vi "Post action.vi"(6 "Index":i32=41, 8 "error in (no error)":errorcluster, 9 "PostAction":T1, 11 "SweepControl":refnum<class "SMO.SweepControl.lvclass">) -> (0 "error out":errorcluster, 3 "SweepControl":refnum<class "SMO.SweepControl.lvclass">)   [LabVIEW 2019, in "SMO.SweepControl.lvclass"]
uses:
  SMO.SweepControl.lvclass
  <userlib>/LevyLab/Instrument Framework/Instrument Types/Cryostat/Instrument.Cryostat.lvclass
  SMO.Control Experiment/SMO.Control Experiment.lvclass
  Control Experiment SM/Control Experiment SM.lvclass
  C:/Program Files (x86)/National Instruments/LabVIEW 2019/user.lib/LevyLab/Instrument Framework/SMOs/Instrument/Instrument.lvclass
  C:/Program Files (x86)/National Instruments/LabVIEW 2019/vi.lib/JKI/JKI SMO/SMO/SMO.lvclass
  Typedefs/Enum - PostAction.ctl
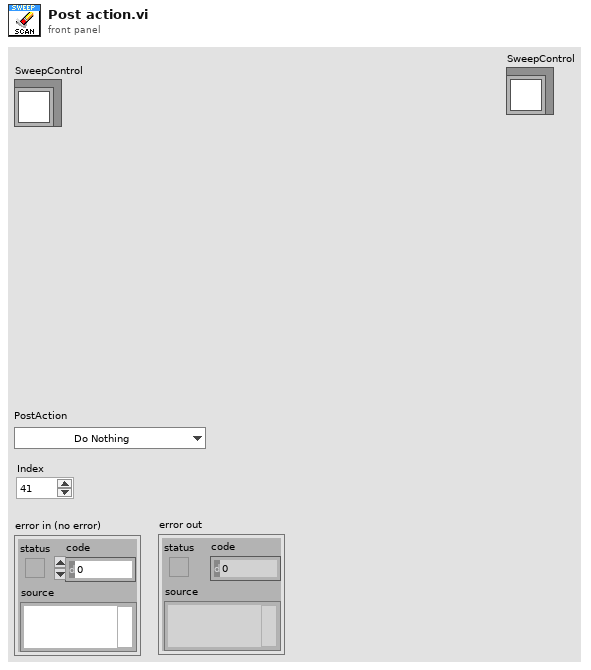
[diagram p1: front panel]
types:
  T1 = typedef "SMO.SweepControl.lvclass/Enum - PostAction.ctl" = enum16{"Do Nothing", "Wait (time)", "Wait (Temperature)", "Wait (<T ; B sweep)", "Wait (Magnet)"}
  T2 = typedef "SMO.SweepControl.lvclass/Cluster - ScanParamters.ctl" = cluster{"Start":dbl, "End":dbl, "Step":dbl, "Rate":dbl, "Waveform type":enum16{"linear", "triangle", "power"}, "wait (ms or K)":dbl, "Address":string, "channel":i32}
  T3 = typedef "SMO.Control Experiment.lvclass/Instruments--cluster.ctl" = cluster{"Lockin":refnum<class "Instrument.Lockin.lvclass">, "Temperature":refnum<class "Instrument.Cryostat.lvclass">, "Magnet":refnum<class "Instrument.Cryostat.lvclass">, "Rotator":refnum<class "Instrument.Cryostat.lvclass">, "Level":refnum<class "Instrument.Cryostat.lvclass">, "C Bridge":refnum<class "Instrument.CBridge.lvclass">, "Optical Delay Line":refnum<class "Instrument.DelayLine.lvclass">, "Strain Cell":refnum<class "Instrument.Strain.lvclass">, "VNA":refnum<class "Instrument.VNA.lvclass">, "Voltage Source":refnum<class "Instrument.VSource.lvclass">, "KH7008":refnum<class "Instrument.KH7008.lvclass">[]}
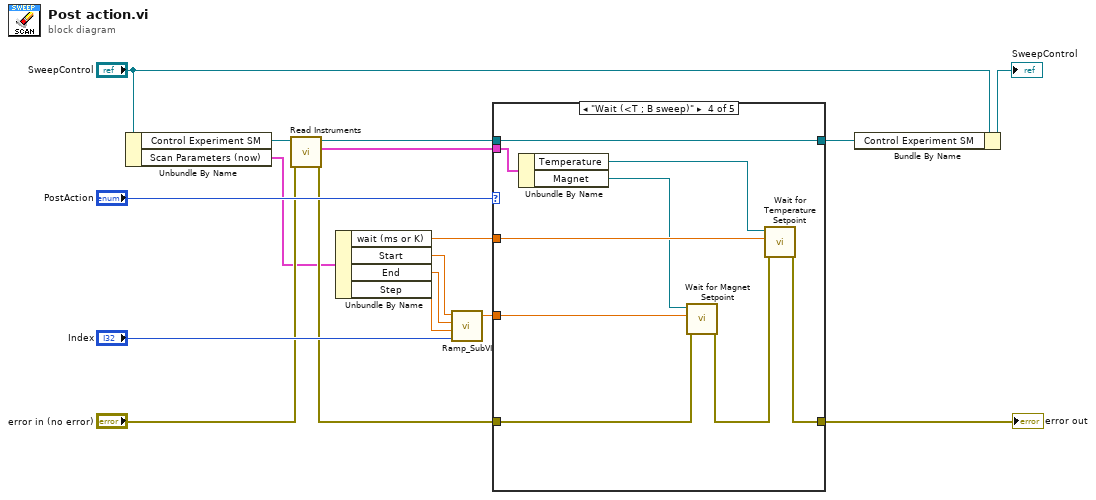
[diagram p0: block diagram]
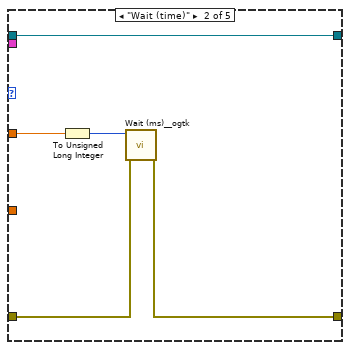
[diagram p3: hidden frame]
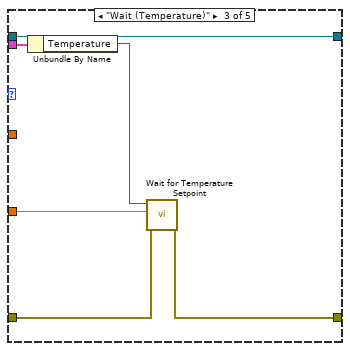
[diagram p4: hidden frame]
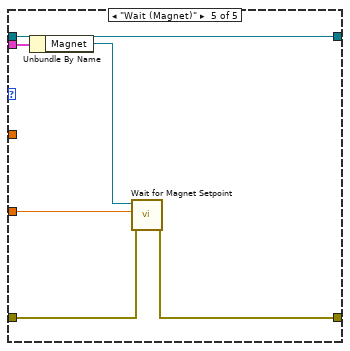
[diagram p5: hidden frame]
diagram:
  n1 = Unbundle By Name("SweepControl") -> ("Control Experiment SM"=w9:refnum<class "Control Experiment SM.lvclass">, "Scan Parameters (now)"=w1:T2)
  n2 = call "Read Instruments.vi"("error in (no error)"="error in (no error)", "Control Experiment"=w9) -> ("error out"=w6:errorcluster, "Instruments"=w8:T3, "Control Experiment out"=w2:refnum<class "SMO.Control Experiment.lvclass">)  [unwired: 7 in]
  n3 = Unbundle By Name(w1) -> ("wait (ms or K)"=w11:dbl, "Start"=w14:dbl, "End"=w13:dbl, "Step"=w12:dbl)
  n4 = call <userlib>:"Ramp_SubVI.vi"("index"="Index", "step"=w12, "end"=w13, "start"=w14) -> ("Numeric"=w16:dbl)  [unwired: 1 in, 1 out]
  n5 = case shown="\"Wait (<T ; B sweep)\"" "PostAction" {
    tunnel: w16 -> [_ _ w30 w34 w45]
    tunnel: w11 -> [_ w24 _ w36 _]
    tunnel: w6 -> [w19 w23 w29 w33 w44]
    tunnel: [w19 w22 w28 w39 w43] -> w10
    tunnel: w8 -> [_ _ w27 w38 w42]
    tunnel: [w18 w21 w25 w35 w40] -> w3
    tunnel: w2 -> [w18 w21 w25 w35 w40]
    frame "Do Nothing", Default {
    }
    frame "Wait (time)" {
      n6 = To Unsigned Long Integer(number=w24) -> (unsigned 32bit integer=w20:u32)
      n7 = call <userlib>:"Wait (ms)__ogtk.vi"("error in (no error)"=w23, "milliseconds to wait"=w20) -> ("error out"=w22:errorcluster)  [unwired: 8 in, 1 out]
    }
    frame "Wait (Temperature)" {
      n8 = Unbundle By Name(w27) -> ("Temperature"=w26:refnum<class "Instrument.Cryostat.lvclass">)
      n9 = call <userlib>:"Wait for Temperature Setpoint.vi"("error in (no error)"=w29, "Setpoint (K)"=w30, "Instrument.Cryostat in"=w26) -> ("error out"=w28:errorcluster)  [unwired: 7 in, 1 out]
    }
    frame "Wait (<T ; B sweep)" {
      n10 = Unbundle By Name(w38) -> ("Temperature"=w37:refnum<class "Instrument.Cryostat.lvclass">, "Magnet"=w31:refnum<class "Instrument.Cryostat.lvclass">)
      n11 = call <userlib>:"Wait for Magnet Setpoint.vi"("error in (no error)"=w33, "Setpoint (T)"=w34, "Instrument.Cryostat in"=w31) -> ("error out"=w32:errorcluster)  [unwired: 7 in, 1 out]
      n12 = call <userlib>:"Wait for Temperature Setpoint.vi"("error in (no error)"=w32, "Setpoint (K)"=w36, "Instrument.Cryostat in"=w37) -> ("error out"=w39:errorcluster)  [unwired: 7 in, 1 out]
    }
    frame "Wait (Magnet)" {
      n13 = Unbundle By Name(w42) -> ("Magnet"=w41:refnum<class "Instrument.Cryostat.lvclass">)
      n14 = call <userlib>:"Wait for Magnet Setpoint.vi"("error in (no error)"=w44, "Setpoint (T)"=w45, "Instrument.Cryostat in"=w41) -> ("error out"=w43:errorcluster)  [unwired: 7 in, 1 out]
    }
  }
  "error out" <- w10
  n15 = Bundle By Name(cluster="SweepControl", "Control Experiment SM"=w3) -> (→"SweepControl":refnum<class "SMO.SweepControl.lvclass">)
